vi "Read Ring Text.vi"(9 "NamedNumeric in":refnum<class "NamedNumeric.lvclass">) -> (3 "NamedNumeric out":refnum<class "NamedNumeric.lvclass">, 4 "Ring Text":refnum<class "Text.lvclass">)   [LabVIEW 2014, in "NamedNumeric.lvclass"]
uses:
  NamedNumeric.lvclass
  Text/Text.lvclass
  NamedNumeric.lvclass/NamedNumeric.ctl
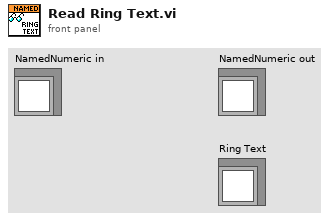
[diagram p1: front panel]
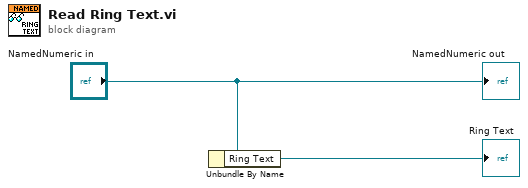
[diagram p0: block diagram]
diagram:
  n1 = Unbundle By Name("NamedNumeric in") -> ("Ring Text"=→"Ring Text":refnum<class "Text.lvclass">)
  "NamedNumeric out" <- "NamedNumeric in"
